vi "Error Channels Write Array.vi"(8 "error in":errorcluster, 9 "Number of Channels":u32, 10 "Value to Write":i32, 11 "Power Supply In":refnum<class "Power Supply.lvclass">) -> (0 "error out":errorcluster, 3 "Power Supply Out":refnum<class "Power Supply.lvclass">)   [LabVIEW 2023, in "Power Supply.lvclass"]
uses:
  Power Supply.lvclass
  Power Supply.lvclass/Power Supply.ctl
  Low Level Capabilities/Error Channels/Error Channels.lvclass
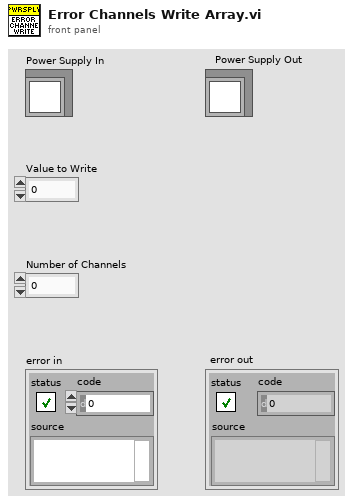
[diagram p1: front panel]
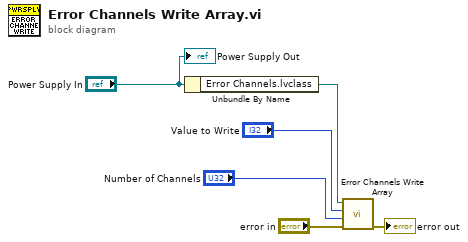
[diagram p0: block diagram]
diagram:
  n1 = Unbundle By Name("Power Supply In") -> ("Error Channels.lvclass"=w6:refnum<class "Error Channels.lvclass">)
  n2 = call-dynamic "Error Channels Write Array.vi"("error in (no error)"="error in", "Number of Channels"="Number of Channels", "Value to Write"="Value to Write", "Error Channels in"=w6) -> ("error out"=→"error out":errorcluster)  [unwired: 6 in, 1 out]
  "Power Supply Out" <- "Power Supply In"
